vi "Multi-Function-Synch AI-AO_LEV.vi"() -> ()   [LabVIEW 2013]
doc: "I. Description:\nThis example demonstrates how to continuously acquire and generate data at the same time, synchronized with one another.\n\nII. Instructions for Running:\n1. Select the physical channel to correspond to where your signal is input on the DAQ device. Also, select the corresponding channel for where your signal is being generated.\n2. Enter the minimum and maximum voltage ranges.\nNote: For better accuracy try to match the input range to the expected voltage level of the measured signal.\n3. Set the sample rate of the acquisition.\nNote: The rate should be at least twice as fast as the maximum frequency component of the signal being acquired. \n6. Select the Rate for the generation\n7. Select what type of signal to generate and the amplitude.\nNote: This example requires two DMA channels to run. If your hardware does not support two DMA channels, you need to set the Data Transfer Mechanism property for the Analog Output Task to use \"Interrupts\". The Data Transfer Mechanism property is located in the DAQmx Channel Property hierarchy at:\n\nDAQmx Channel Property Node>>Analog Output>>General Properties>>Advanced>>Data Transfer and Memory>>Data Transfer Mechanism\n\nRefer to your device documentation to determine how many DMA channels are supported for your hardware.\n\nIII. Block Diagram Steps:\n1. Create an analog input voltage channel. Also, create an analog output voltage channel.\n2. Set the rate for the sample clock. Additionally, define the sample mode to be continuous. Also, set the sample clock rate for the signal generation.\n2a. Call the Get Terminal Name with Device Prefix VI. This will take a Task and a terminal and create a properly formatted device + terminal name to use as the source of the Trigger.\n3. Define the parameters for a Digital Edge Start Trigger. Set the Analog output to trigger off the AI Start Trigger. This is an internal trigger signal.\n4. Use the Basic Function Generator VI to create the signal to be generated.\n5. Call the Start VI to arm the two functions. Make sure the analog output is armed before the analog input. This will ensure both will start at the same time.\n6. Read the waveform data in a loop until the user hits the stop button or an error occurs. The Is Task Done? VI is used to check for errors in the Analog Output Task.\n7. Call the Clear VI to Clear the Task\n8. Use the popup dialog box to display an error if any.\n\nIV. I/O Connections Overview:\nMake sure your signal input/output terminals match the Physical Channel I/O controls."
uses:
  <vilib>/Utility/error.llb/DialogType.ctl
  <vilib>/DAQmx/write.llb/DAQmx Write (Analog Wfm 1Chan NSamp).vi
  <vilib>/DAQmx/read.llb/DAQmx Read (Analog Wfm 1Chan NSamp).vi
  <vilib>/DAQmx/create/channels.llb/DAQmx Create Channel (AI-Voltage-Basic).vi
  <vilib>/DAQmx/configure/timing.llb/DAQmx Timing (Sample Clock).vi
  <vilib>/DAQmx/create/channels.llb/DAQmx Create Channel (AO-Voltage-Basic).vi
  <vilib>/DAQmx/configure/trigger.llb/DAQmx Start Trigger (Digital Edge).vi
  <vilib>/Utility/file.llb/Write To Spreadsheet File (DBL).vi
  <vilib>/DAQmx/miscellaneous.llb/DAQmx Fill In Error Info.vi
  <vilib>/measure/NI_MABase.lvlib
  <resource>/objmgr/daqmx.rc
panel:
  in  "file path (dialog if empty)":path
  out "Actual Update Generation Rate":dbl=5000.0 format="%0.2f"
  out "Actual Input Rate":dbl=10000.0 format="%0.2f"
  in  "Amplitude":dbl=1.0 format="%0.2p"
  in  "Signal Type":T1(ring)
  in  "rate":dbl=5000.0 caption="Update Generation Rate" format="%0.2f"
  in  "Samples to Read":i32=1000
  in  "minimum value":dbl=-10.0 caption="Output Minimum Value" format="%0.2f"
  in  "maximum value":dbl=10.0 caption="Output Maximum Value" format="%0.2f"
  in  "physical channels":tag="Dev1/ao0" caption="Output Physical Channels"
  in  "Maximum Value":dbl=10.0 caption="Input Maximum Value" format="%0.2f"
  in  "Minimum Value":dbl=-10.0 caption="Input Minimum Value" format="%0.2f"
  in  "Physical Channel":tag="Dev1/ai0" caption="Input Physical Channel"
  in  "Rate":dbl=10000.0 caption="Input Rate" format="%0.2f"
  in  "stop":bool
  out "Measurement":waveform(dbl)[](graph)
  # "For instructions, select Help>>Show Context Help"
  # "Channel Parameters"
  # "Timing Parameters"
  # "Signal Generation"
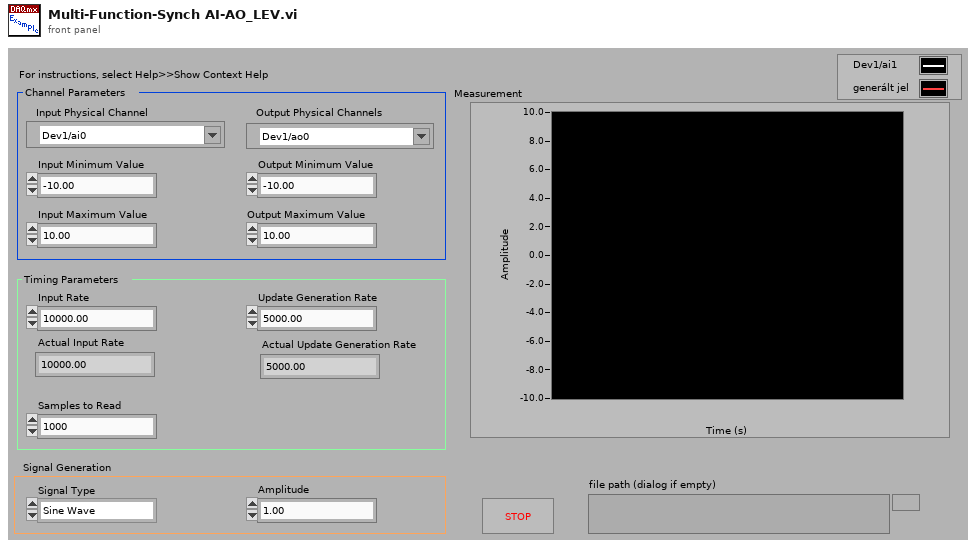
[diagram p1: front panel]
types:
  T1 = enum16{"Sine Wave", "Triangle Wave", "Square Wave", "Sawtooth Wave"}
  T2 = typedef "DialogType.ctl" = u16
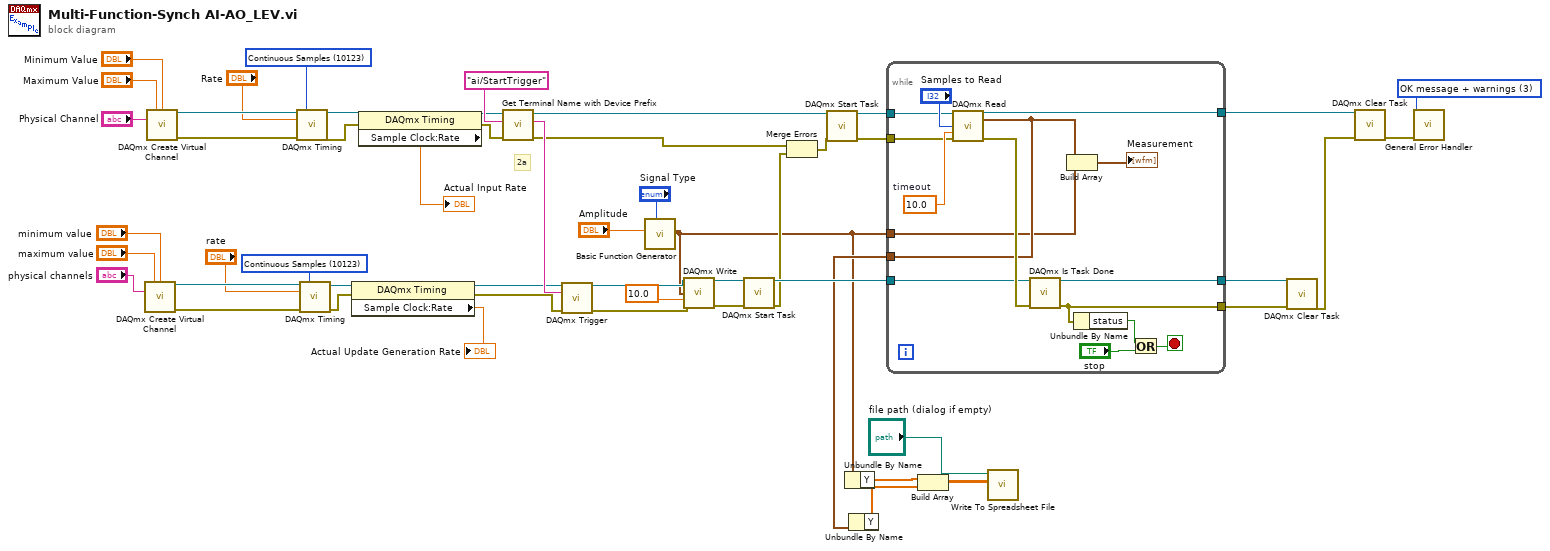
[diagram p0: block diagram]
diagram:
  w31 = T2 3 items=["no dialog", "OK message", "continue or stop message", "OK message + warnings", "continue/stop + warnings"] ("type of dialog (OK msg:1)")
  w43 = 10123 items=["Finite Samples"=10178, "Continuous Samples"=10123] ("sample mode")
  w49 = 10123 items=["Finite Samples"=10178, "Continuous Samples"=10123] ("sample mode")
  # "2a"
  n1 = call-poly <vilib>:"DAQmx Create Virtual Channel.vi"("maximum value"="maximum value", "minimum value"="minimum value", "physical channels"="physical channels") -> ("task out"=w42:refnum<k21>, "error out"=w41:errorcluster)  [unwired: 11 in]
  n2 = call-poly <vilib>:"DAQmx Create Virtual Channel.vi"("maximum value"="Maximum Value", "minimum value"="Minimum Value", "physical channels"="Physical Channel") -> ("task out"=w47:refnum<k21>, "error out"=w48:errorcluster)  [unwired: 11 in]
  n3 = call-poly <vilib>:"DAQmx Timing.vi"("task/channels in"=w47, "sample mode"=w49, "rate"="Rate", "error in"=w48) -> ("task out"=w14:refnum<k21>, "error out"=w13:errorcluster)  [unwired: 10 in]
  n4 = call-poly <vilib>:"DAQmx Timing.vi"("task/channels in"=w42, "sample mode"=w43, "rate"="rate", "error in"=w41) -> ("task out"=w24:refnum<k21>, "error out"=w23:errorcluster)  [unwired: 10 in]
  n5 = property class="DAQmx Timing"(reference=w24, error in=w23) -> (reference out=w25:refnum<k21>, error out=w22:errorcluster, "Sample Clock:Rate"=→"Actual Update Generation Rate":dbl)
  n6 = property class="DAQmx Timing"(reference=w14, error in=w13) -> (reference out=w12:refnum<k21>, error out=w11:errorcluster, "Sample Clock:Rate"=→"Actual Input Rate":dbl)
  n7 = call "Get Terminal Name with Device Prefix.vi"("error in (no error)"=w11, "Local Terminal Name"="ai/StartTrigger" ("terminal"), "task/channels in"=w12) -> ("error out"=w19:errorcluster, "Terminal Name with Device Prefix"=w26:tag, "task out"=w21:refnum<k21>)  [unwired: 6 in]
  n8 = call-poly <vilib>:"DAQmx Trigger.vi"("task/channels in"=w25, "source"=w26, "error in"=w22) -> ("task out"=w33:refnum<k21>, "error out"=w34:errorcluster)  [unwired: 11 in]
  n9 = call <vilib>:"Basic Function Generator.vi"("signal type"="Signal Type", "amplitude"="Amplitude") -> ("signal out"=w1:waveform(dbl))  [unwired: 7 in, 2 out]
  n10 = call-poly <vilib>:"DAQmx Write.vi"("task/channels in"=w33, "data"=w1, "timeout"=10.0 ("Wirite Timeout"), "error in"=w34) -> ("task out"=w36:refnum<k21>, "error out"=w35:errorcluster)  [unwired: 9 in, 1 out]
  n11 = call <vilib>:"DAQmx Start Task.vi"("task/channels in"=w36, "error in"=w35) -> ("task out"=w40:refnum<k21>, "error out"=w18:errorcluster)  [unwired: 12 in]
  n12 = Merge Errors(w19, w18) -> (w17:errorcluster)
  n13 = call <vilib>:"DAQmx Start Task.vi"("task/channels in"=w21, "error in"=w17) -> ("task out"=w20:refnum<k21>, "error out"=w16:errorcluster)  [unwired: 12 in]
  n14 = Unbundle By Name(w1) -> ("Y"=w5:dbl[])
  n15 = while {
    tunnel: [w67] -> w50
    tunnel: w40 -> [w60]
    tunnel: [w59] -> w39
    tunnel: w20 -> [w58]
    tunnel: w16 -> [w57]
    tunnel: [w56] -> w9
    tunnel: [w55] -> w6
    tunnel: w1 -> [w54]
    stop <- w65 stop-if-true
    w66 = 10.0  # timeout
    n16 = call-poly <vilib>:"DAQmx Read.vi"("task/channels in"=w58, "number of samples per channel"="Samples to Read", "timeout"=w66, "error in"=w57) -> ("task out"=w67:refnum<k21>, "data"=w55:waveform(dbl), "error out"=w61:errorcluster)  [unwired: 9 in]
    n17 = call <vilib>:"DAQmx Is Task Done.vi"("task/channels in"=w60, "error in"=w61) -> ("task out"=w59:refnum<k21>, "error out"=w56:errorcluster)  [unwired: 11 in, 1 out]
    n18 = Build Array(w55, w54) -> (→"Measurement":waveform(dbl)[])
    n19 = Unbundle By Name(w56) -> ("status"=w62:bool)
    n20 = Or(x=w62, y="stop") -> (x .or. y?=w65:bool)
  }
  n21 = Unbundle By Name(w6) -> ("Y"=w4:dbl[])
  n22 = Build Array(w5, w4) -> (w3:dbl[][])
  n23 = call-poly <vilib>:"Write To Spreadsheet File.vi"("2D data"=w3, "file path (dialog if empty)"="file path (dialog if empty)") -> ()  [unwired: 6 in, 1 out]
  n24 = call <vilib>:"DAQmx Clear Task.vi"("task in"=w39, "error in"=w9) -> ("error out"=w8:errorcluster)  [unwired: 13 in]
  n25 = call <vilib>:"DAQmx Clear Task.vi"("task in"=w50, "error in"=w8) -> ("error out"=w7:errorcluster)  [unwired: 13 in]
  n26 = call <vilib>:"General Error Handler.vi"("type of dialog (OK msg:1)"=w31, "error in (no error)"=w7) -> ()  [unwired: 9 in, 5 out]
